vi "Update MCP Server.vi"() -> ()   [LabVIEW 2025, in "Tools.lvlib"]
uses:
  Tools.lvlib
  Server Creator Data.ctl
  MCP Creator States.ctl
  PyServer/PyServer.lvclass
panel:
  in  "Tab Control":enum32{"Configuration", "Python Code"}(tab)
  in  "Load Config":bool
  in  "Save Config":bool
  in  "Library Path":path
  in  "Remove Tool":bool
  in  "Description":string
  in  "Tools":i32[](listbox)
  in  "Add_Tool":bool
  in  "Add Folder":bool
  out "Python String":string
  in  "error in (no error)":errorcluster
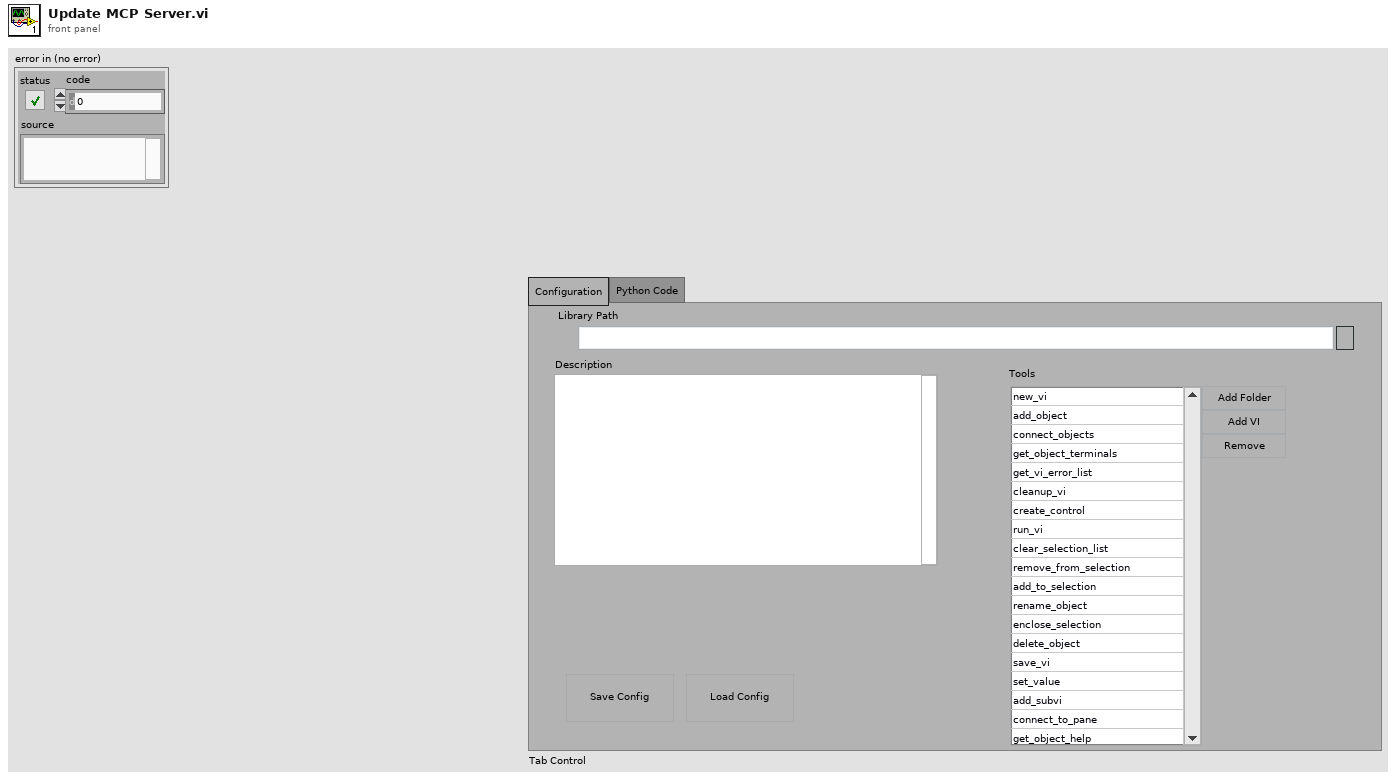
[diagram p1: front panel]
types:
  T1 = typedef "Tools.lvlib/MCP Creator States.ctl" = enum16{"Wait For Event", "Update UI", "Update Server", "Load Project"}
  T2 = typedef "Tools.lvlib/Server Creator Data.ctl" = cluster{"Name":string, "Description":string, "Tools":path[], "Project Path":path}
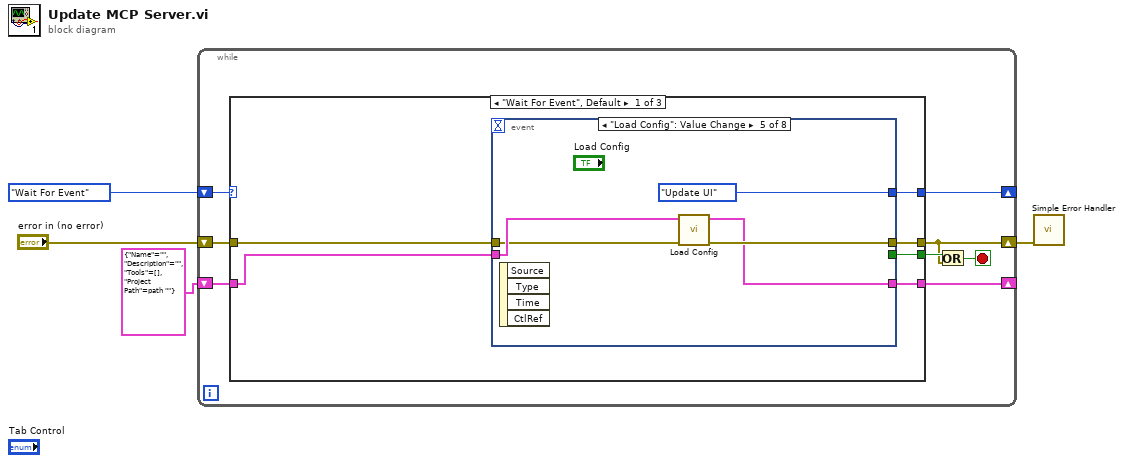
[diagram p0: block diagram]
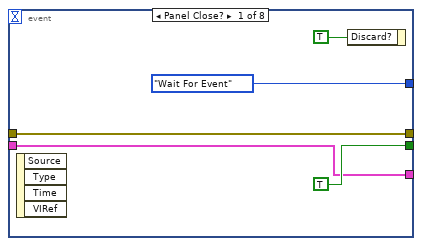
[diagram p2: hidden frame]
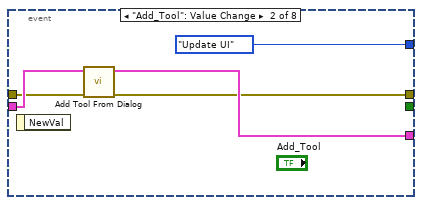
[diagram p3: hidden frame]
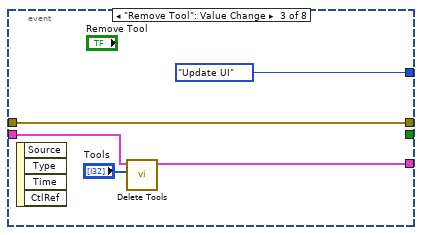
[diagram p4: hidden frame]
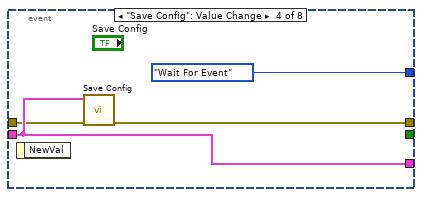
[diagram p5: hidden frame]
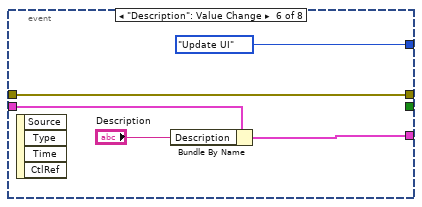
[diagram p6: hidden frame]
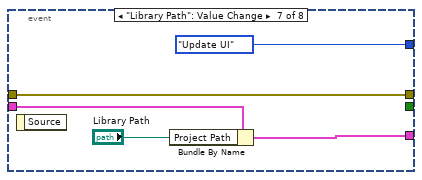
[diagram p7: hidden frame]
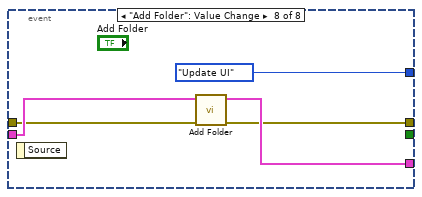
[diagram p8: hidden frame]
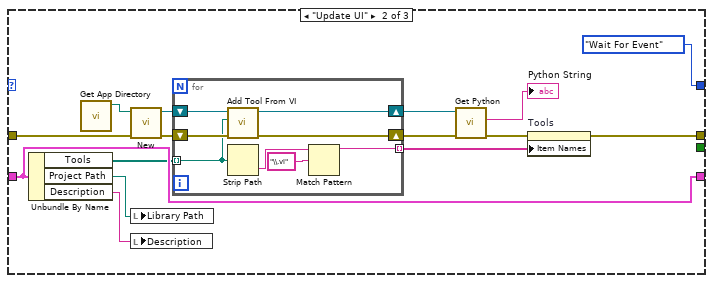
[diagram p9: hidden frame]
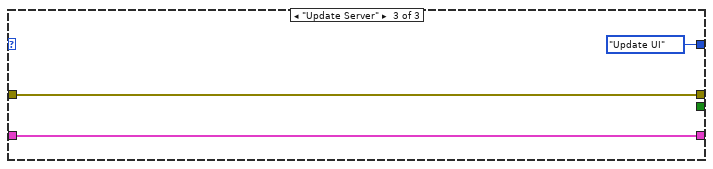
[diagram p10: hidden frame]
diagram:
  n1 = while {
    shift-right: [w12] -> _
    shift-left: T2 {"Name"="", "Description"="", "Tools"=[], "Project Path"=path ""} -> [w11]
    shift-right: [w7] -> w2
    shift-left: "error in (no error)" -> [w10]
    shift-right: [w5] -> _
    shift-left: MCP_Creator_States."Wait For Event" -> [w6]
    stop <- w8 stop-if-true
    n2 = case shown="\"Wait For Event\", Default" w6 {
      tunnel: [w18 w64 w83] -> w12
      tunnel: w11 -> [w17 w64 w83]
      tunnel: w10 -> [w16 w65 w82]
      tunnel: [w15 _ _] -> w9
      tunnel: [w14 w60 w82] -> w7
      tunnel: [w13 MCP_Creator_States."Wait For Event" MCP_Creator_States."Update UI"] -> w5
      frame "Wait For Event", Default {
        n3 = event shown="[4] \"Load Config\": Value Change" {
          selector: _ -> [_ _ _ _ _ _ _ _]
          dyn-events: _ -> [_ _ _ _ _ _ _ _]
          timeout: _ -> [_ _ _ _ _ _ _ _]
          tunnel: [TRUE ("Discard?") _ _ _ _ _ _ _] -> w15
          tunnel: [w20 w28 w31 w37 w39 w44 w50 w56] -> w18
          tunnel: w17 -> [w20 w27 w30 w37 w42 w47 w52 w57]
          tunnel: w16 -> [w21 w26 w33 w35 w41 w46 w51 w53]
          tunnel: [w21 w25 w33 w36 w40 w46 w51 w54] -> w14
          tunnel: [MCP_Creator_States."Wait For Event" MCP_Creator_States."Update UI" MCP_Creator_States."Update UI" MCP_Creator_States."Wait For Event" MCP_Creator_States."Update UI" MCP_Creator_States."Update UI" MCP_Creator_States."Update UI" MCP_Creator_States."Update UI"] -> w13
          event Panel Close? {
            n4 = event-data() -> ()  [unwired: 1 in, 4 out]
            n5 = event-data("Discard?"=TRUE) -> ()  [unwired: 1 in, 1 out]
          }
          event "Add_Tool": Value Change {
            n6 = event-data() -> ()  [unwired: 1 in, 1 out]
            n7 = call "Add Tool From Dialog.vi"("error in (no error)"=w26, "Server Creator Data in"=w27) -> ("error out"=w25:errorcluster, "Server Creator Data out"=w28:T2)  [unwired: 8 in]
          }
          event "Remove Tool": Value Change {
            n8 = event-data() -> ()  [unwired: 1 in, 4 out]
            n9 = call "Delete Tools.vi"("Tools"="Tools", "Server Creator Data in"=w30) -> ("Server Creator Data out"=w31:T2)  [unwired: 9 in]
          }
          event "Save Config": Value Change {
            n10 = event-data() -> ()  [unwired: 1 in, 1 out]
            n11 = call "Save Config.vi"("error in (no error)"=w35, "Server Creator Data"=w37) -> ("error out"=w36:errorcluster)  [unwired: 9 in]
          }
          event "Load Config": Value Change {
            n12 = event-data() -> ()  [unwired: 1 in, 4 out]
            n13 = call "Load Config.vi"("error in (no error)"=w41, "Server Creator Data in"=w42) -> ("error out"=w40:errorcluster, "Server Creator Data out"=w39:T2)  [unwired: 8 in]
          }
          event "Description": Value Change {
            n14 = event-data() -> ()  [unwired: 1 in, 4 out]
            n15 = Bundle By Name(cluster=w47, "Description"="Description") -> (w44:T2)
          }
          event "Library Path": Value Change {
            n16 = event-data() -> ()  [unwired: 1 in, 1 out]
            n17 = Bundle By Name(cluster=w52, "Project Path"="Library Path") -> (w50:T2)
          }
          event "Add Folder": Value Change {
            n18 = event-data() -> ()  [unwired: 1 in, 1 out]
            n19 = call "Add Folder.vi"("error in (no error)"=w53, "Server Creator Data in"=w57) -> ("error out"=w54:errorcluster, "Server Creator Data out"=w56:T2)  [unwired: 8 in]
          }
        }
      }
      frame "Update UI" {
        n20 = Unbundle By Name(w64) -> ("Tools"=w63:path[], "Project Path"=w59:path, "Description"=w58:string)
        n21 = call "Get App Directory.vi"() -> ("appended path"=w67:path)  [unwired: 11 in]
        n22 = call "New.vi"("error in (no error)"=w65, "Server Path"=w67) -> ("error out"=w70:errorcluster, "PyServer out"=w68:refnum<class "PyServer.lvclass">)  [unwired: 8 in]
        n23 = local write "Library Path"(w59) -> ()
        n24 = local write "Description"(w58) -> ()
        n25 = for {
          tunnel: w63 -> [w76] mode=indexing
          shift-right: [w79] -> w66
          shift-left: w70 -> [w80]
          shift-right: [w77] -> w69
          shift-left: w68 -> [w78]
          tunnel: [w73] -> w62 mode=indexing
          n26 = call "Add Tool From VI.vi"("error in (no error)"=w80, "vi path"=w76, "PyServer in"=w78) -> ("error out"=w79:errorcluster, "PyServer out"=w77:refnum<class "PyServer.lvclass">)  [unwired: 7 in]
          n27 = Strip Path(path=w76) -> (name=w75:string)  [unwired: 1 out]
          n28 = Match Pattern(string=w75, regular expression="\\.vi") -> (before substring=w73:string)  [unwired: 1 in, 3 out]
        }
        n29 = call "Get Python.vi"("error in (no error)"=w66, "PyServer in"=w69) -> ("error out"=w61:errorcluster, "resulting string"=→"Python String":string)  [unwired: 7 in, 1 out]
        n30 = property on="Tools" class="LstBox (strict)"(error in=w61, "Item Names"=w62) -> (error out=w60:errorcluster)  [unwired: 1 in, 1 out]
      }
      frame "Update Server" {
      }
    }
    n31 = Or(x=w9, y=w7) -> (x .or. y?=w8:bool)
  }
  n32 = call <vilib>:"Simple Error Handler.vi"("error in (no error)"=w2) -> ()  [unwired: 4 in, 5 out]
